vi "Create image name.vi"(8 "error in (no error)":errorcluster, 9 "Suffix":string, 10 "Channel":u8, 11 "Simulated_CCD_Camera in":refnum<class "Simulated Camera.lvclass">) -> (0 "error out":errorcluster, 3 "Simulated_CCD_Camera out":refnum<class "Simulated Camera.lvclass">)   [LabVIEW 2018]
doc: "Create the image name\n\nThis name is composed by the following parts. First, there are the year, month, and day of the beginning of the night in the format YYYYMMDD. Second, there is the string s4cx, where x is the number of the channel. Then, there is the image index in the format 000000. This index is incremented after each acquisition. Finally, there is the suffix provided by the user. Following, there is an example of the image name\n\n20230101_s4c1_000001_zero.fits"
uses:
  Simulated Camera.lvclass
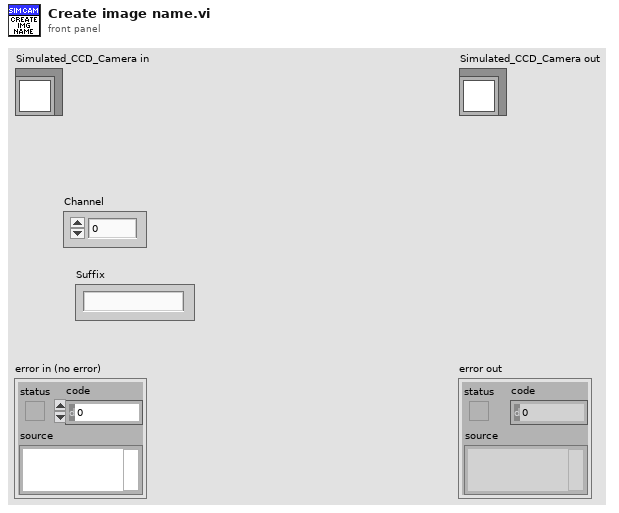
[diagram p1: front panel]
types:
  T1 = typedef "LVDateTimeRec.ctl" = cluster{"fractional second":dbl, "second":i32, "minute":i32, "hour":i32, "day of month":i32, "month":i32, "year":i32, "day of week":i32, "day of year":i32, "DST":i32}
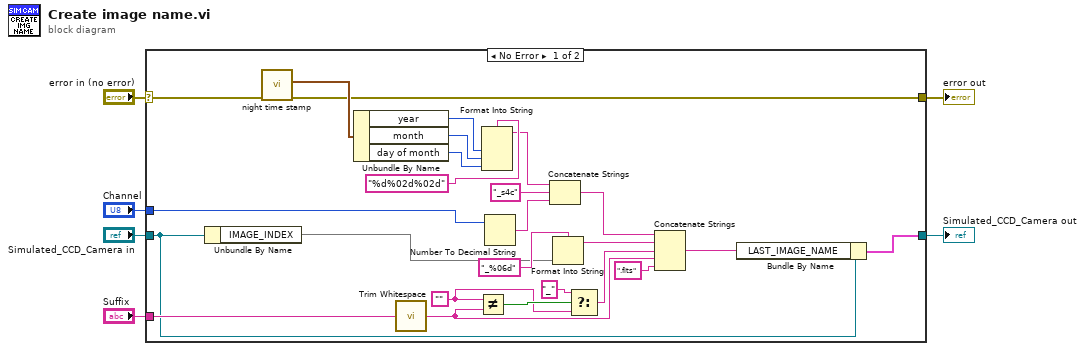
[diagram p0: block diagram]
diagram:
  n1 = case shown="No Error" "error in (no error)" {
    selector: "error in (no error)" -> [w7 w33]
    tunnel: [w8 w33] -> w5
    tunnel: [w21 w32] -> w3
    tunnel: "Simulated_CCD_Camera in" -> [w22 w32]
    tunnel: "Suffix" -> [w24 _]
    tunnel: "Channel" -> [w23 _]
    frame No Error {
      w18 = ""
      n2 = Unbundle By Name(w22) -> ("IMAGE_INDEX"=w10)
      n3 = call "night time stamp.vi"("error in (no error)"=w7) -> ("error out"=w8:errorcluster, "date time rec"=w9:T1)  [unwired: 9 in]
      n4 = Unbundle By Name(w9) -> ("year"=w17:i32, "month"=w16:i32, "day of month"=w11:i32)
      n5 = call <vilib>:"Trim Whitespace.vi"("string"=w24) -> ("trimmed string"=w14:string)  [unwired: 1 in]
      n6 = Not Equal?(x=w18, y=w14) -> (x != y?=w28:bool)
      n7 = Format Into String(format string="%d%02d%02d", w17, w16, w11) -> (resulting string=w19:string)  [unwired: 2 in, 1 out]
      n8 = Number To Decimal String(number=w23) -> (decimal integer string=w30:string)  [unwired: 1 in]
      n9 = Concatenate Strings(w19, "_s4c" ("string"), w30) -> (w29:string)
      n10 = Format Into String(format string="_%06d", w10) -> (resulting string=w13:string)  [unwired: 2 in, 1 out]
      n11 = Select(t="_" ("string"), s=w28, f=w18) -> (s? t:f=w12:string)
      n12 = Concatenate Strings(w29, w13, w12, w14, ".fits" ("string")) -> (w15:string)
      n13 = Bundle By Name(cluster=w22, "LAST_IMAGE_NAME"=w15) -> (w21:cluster{})
    }
    frame Error {
    }
  }
  "error out" <- w5
  "Simulated_CCD_Camera out" <- w3
